vi "io.command-parser.AI.vi"(8 "error in":errorcluster, 10 "Reponse in":string="{ß\u0005\u0001\u0016\u0010\u0001\u0004\u0002ß}", 11 "IoConf in":T1={"ADDR"=0, "Label"="", "Type"=enum."DI", "Mode"=enum."RIO", "Value"="", "Tags"="", "calibration"=[]} {"calibration"."Y" format="%#.3f"; "calibration"."X" format="%#.3f"; "ADDR" format="%04d"}) -> (0 "error out":errorcluster, 1 "AI uncalib out":u16, 2 "AI out":dbl=1.0)   [LabVIEW 2024]
uses:
  controls/IONode.ctl
  controls/type.address.ctl
  controls/enum.io.type.ctl
  controls/enum.io.mode.ctl
  controls/typeXyPoint.ctl
panel:
  out "*(type *) &x 2":string
  out "*(type *) &x":u16
  # "\\DF\\05\\01\\16\\10\\01\\04\\02\\DF"
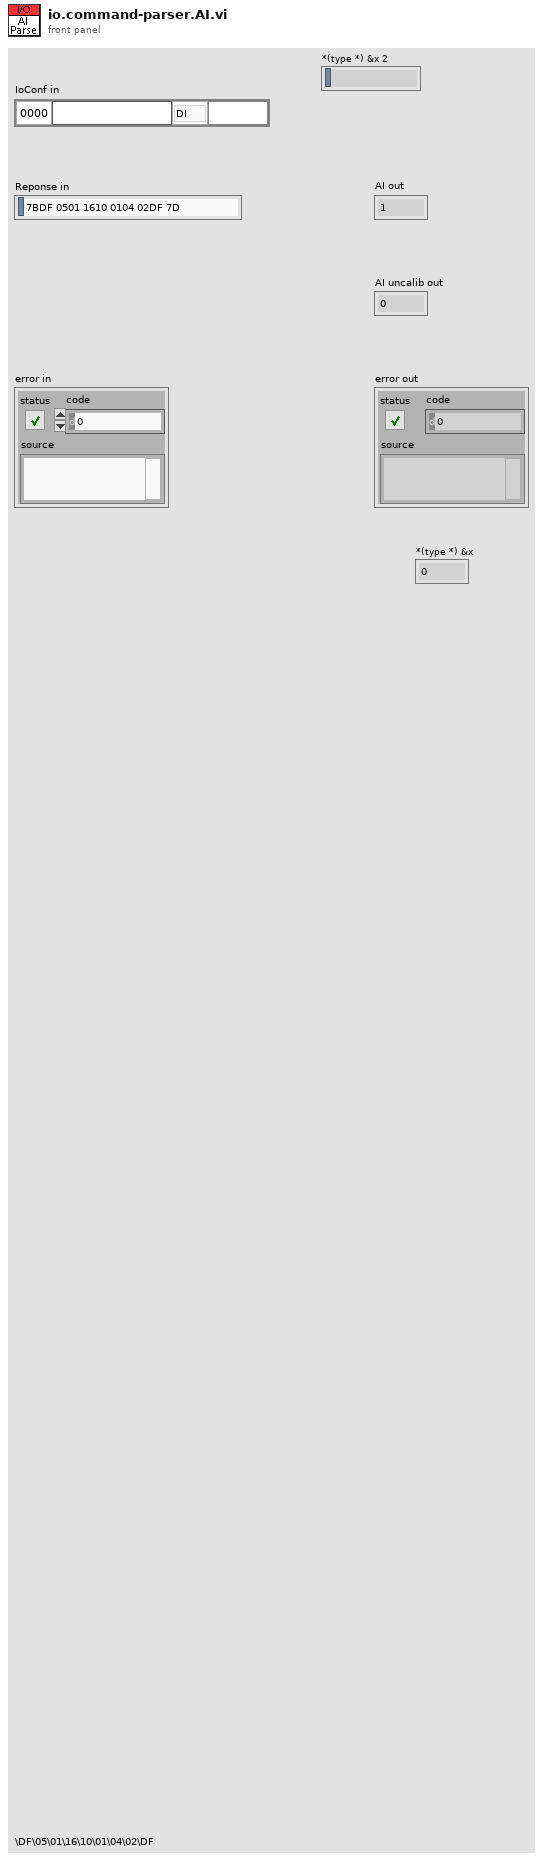
[diagram p1: front panel]
types:
  T1 = typedef "IONode.ctl" = cluster{"ADDR":T2, "Label":string, "Type":T3, "Mode":T4, "Value":string, "Tags":string, "calibration":T5[]}
  T2 = typedef "type.address.ctl" = u16
  T3 = typedef "enum.io.type.ctl" = enum16{"Type", "DI", "DO", "AI", "AO", "VL", "BUF"}
  T4 = typedef "enum.io.mode.ctl" = enum16{"Mode", "RIO", "SIM"}
  T5 = typedef "typeXyPoint.ctl" = cluster{"X":dbl, "Y":dbl}
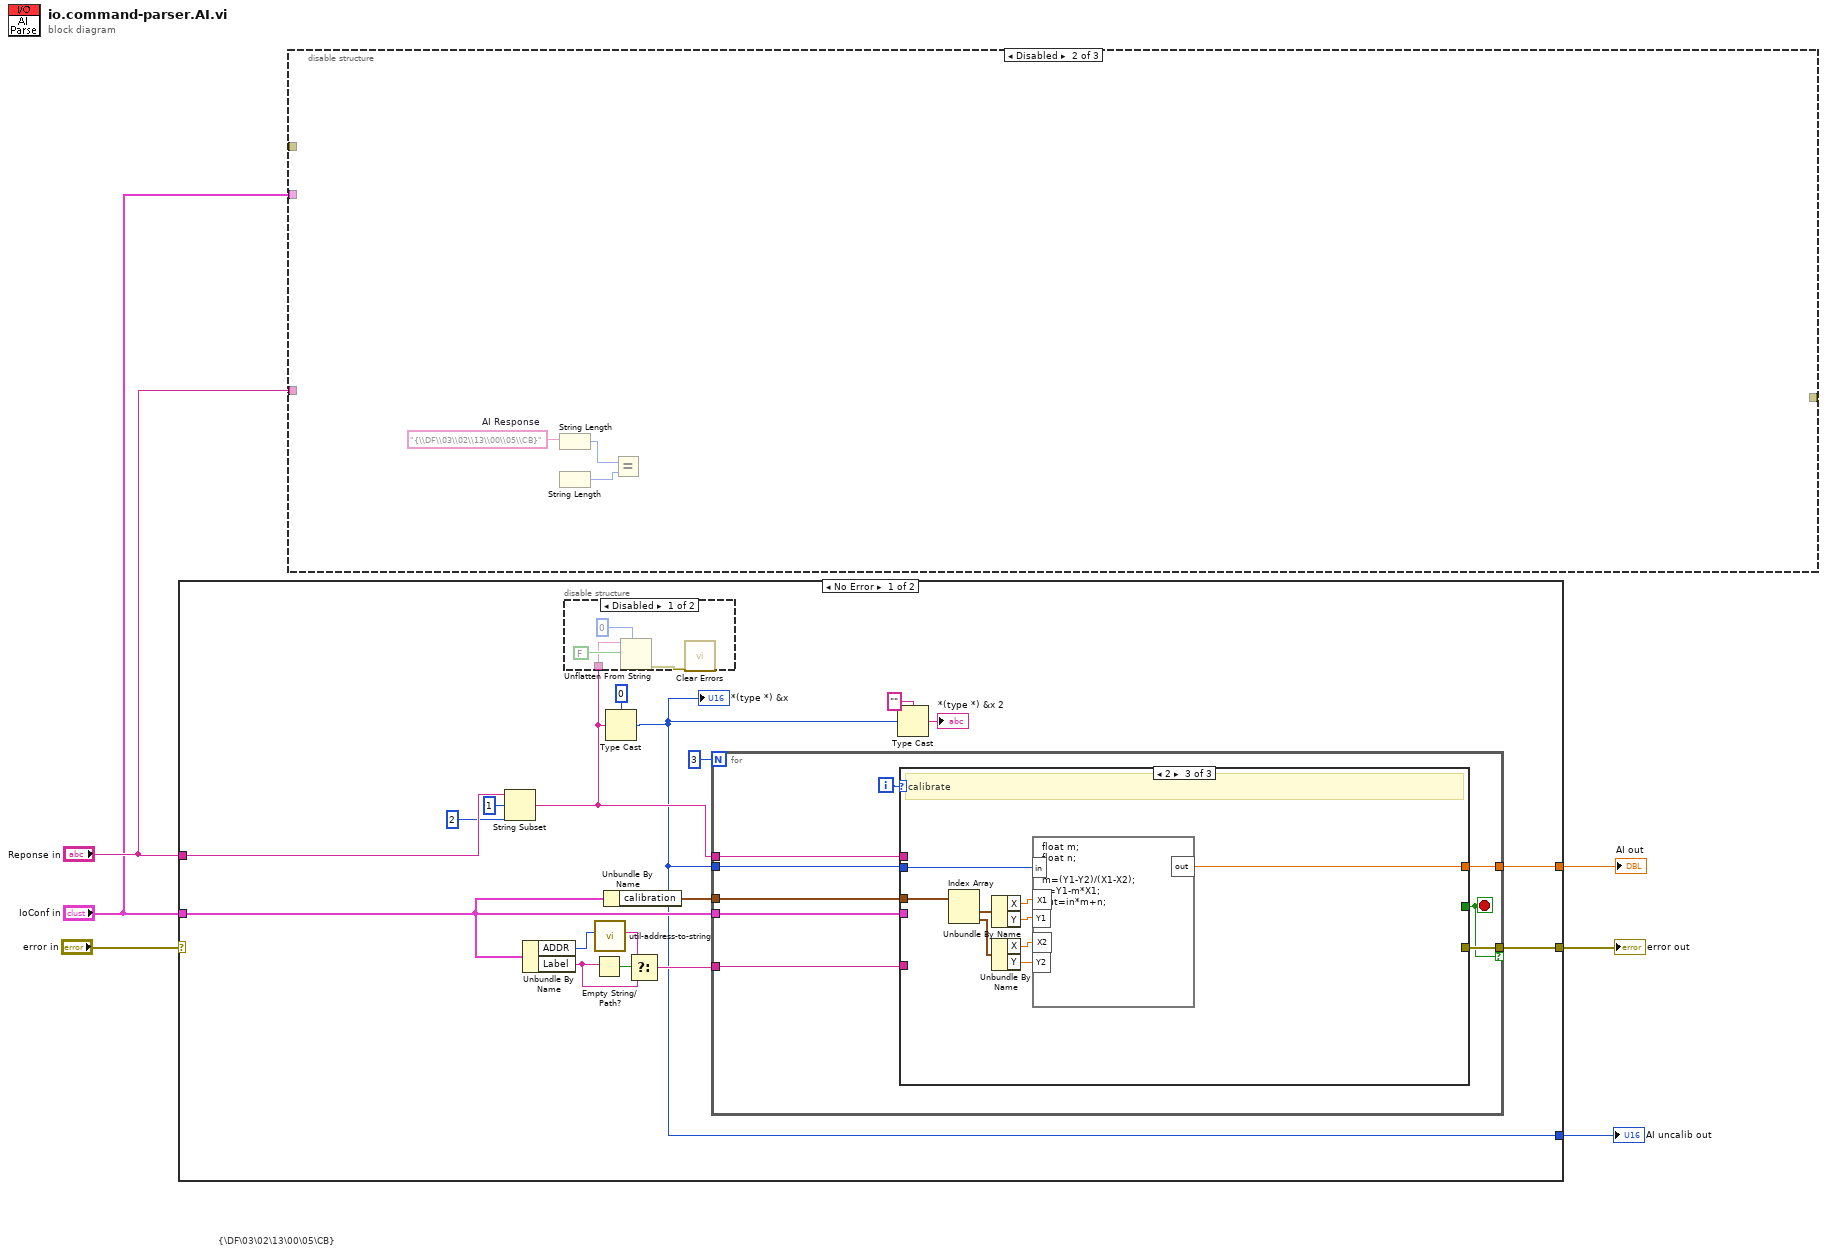
[diagram p0: block diagram]
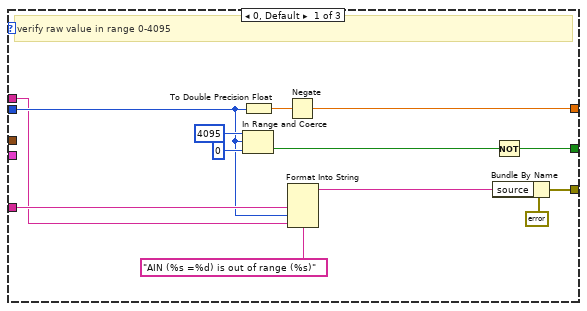
[diagram p3: hidden frame]
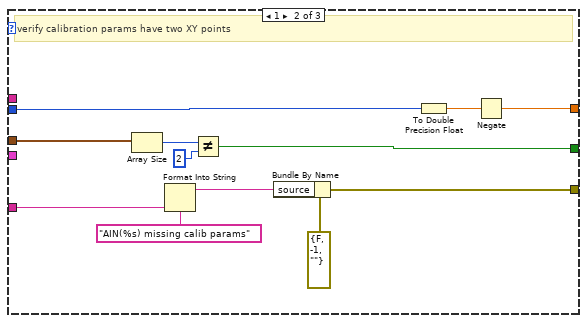
[diagram p4: hidden frame]
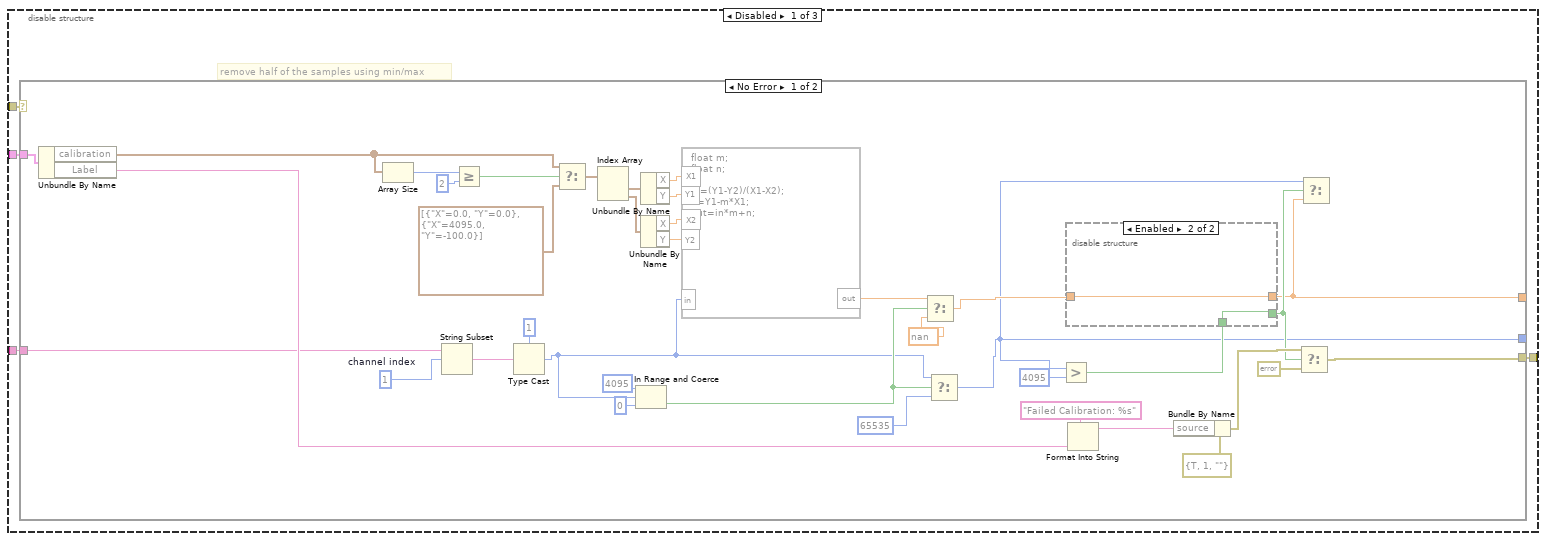
[diagram p6: hidden frame]
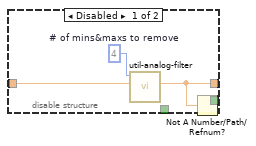
[diagram p7: hidden frame]
diagram:
  # "{\\DF\\03\\02\\13\\00\\05\\CB}"
  n1 = case shown="No Error" "error in" {
    selector: "error in" -> [_ w72]
    tunnel: "Reponse in" -> [w21 _]
    tunnel: "IoConf in" -> [w24 _]
    tunnel: [w23 _] -> w4
    tunnel: [w8 _] -> w3
    tunnel: [w22 w72] -> w2
    frame No Error {
      n2 = String Subset(string=w21, offset (0)=1, length (rest)=2 ("length (rest)")) -> (substring=w9:string)
      n3 = Unbundle By Name(w24) -> ("ADDR"=w19:T2, "Label"=w16:string)
      n4 = disable-structure shown="Disabled" {
        disable-tunnel: w9 -> [w25 _]
        frame Disabled {
          n5 = Unflatten From String(type=u16 0, binary string=w25, data includes array or string size? (T)=FALSE) -> (error out=w26:errorcluster)  [unwired: 2 in, 2 out]
          n6 = call <vilib>:"Clear Errors.vi"("error in (no error)"=w26) -> ()  [unwired: 5 in, 2 out]
        }
        frame Enabled {
        }
      }
      n7 = Empty String/Path?(string/path=w16) -> (empty?=w18:bool)
      n8 = call "util-address-to-string.vi"("ADDR"=w19) -> ("str(ADDR)"=w17:string)  [unwired: 10 in]
      n9 = Unbundle By Name(w24) -> ("calibration"=w13:T5[])
      n10 = Type Cast(type=u16 0, x=w9) -> (*(type *) &x=w8:u16)
      "*(type *) &x" <- w8
      n11 = Select(t=w17, s=w18, f=w16) -> (s? t:f=w15:string)
      n12 = for {
        N: 3 -> [_]
        tunnel: [w36] -> w22 if=w35
        tunnel: w24 -> [w34]
        tunnel: w15 -> [w33]
        tunnel: w8 -> [w32]
        tunnel: w13 -> [w31]
        tunnel: [w30] -> w23
        tunnel: w9 -> [w29]
        i -> [w37]
        stop <- w35 stop-if-true
        n13 = case shown="2" w37 {
          tunnel: [w47 w61 _] -> w35
          tunnel: [w43 w56 _] -> w36
          tunnel: w34 -> [_ _ _]
          tunnel: w33 -> [w42 w59 _]
          tunnel: w32 -> [w39 w51 w64]
          tunnel: w31 -> [_ w55 w65]
          tunnel: [w40 w53 w63] -> w30
          tunnel: w29 -> [w38 _ _]
          frame 0, Default {
            # "verify raw value in range 0-4095"
            n14 = In Range and Coerce(upper limit=u16 4095 ("lower limit"), x=w39, lower limit=u16 0) -> (In Range?=w48:bool)  [unwired: 1 out]
            n15 = To Double Precision Float(number=w39) -> (double precision float=w41:dbl)
            n16 = Negate(x=w41) -> (-x=w40:dbl)
            n17 = Format Into String(format string="AIN (%s =%d) is out of range (%s)", w42, w39, w38) -> (resulting string=w45:string)  [unwired: 2 in, 1 out]
            n18 = Bundle By Name(cluster=errorcluster {"status"=TRUE, "code"=-1, "source"=""} ("error constant"), "source"=w45) -> (w43:errorcluster)
            n19 = Not(x=w48) -> (.not. x?=w47:bool)
          }
          frame 1 {
            # "verify calibration params have two XY points"
            n20 = Array Size(array=w55) -> (size(s)=w52:i32)
            n21 = Format Into String(format string="AIN(%s) missing calib params", w59) -> (resulting string=w57:string)  [unwired: 2 in, 1 out]
            n22 = Not Equal?(x=w52, y=2) -> (x != y?=w61:bool)
            n23 = Bundle By Name(cluster=errorcluster {"status"=FALSE, "code"=-1, "source"=""} ("error constant"), "source"=w57) -> (w56:errorcluster)
            n24 = To Double Precision Float(number=w51) -> (double precision float=w54:dbl)
            n25 = Negate(x=w54) -> (-x=w53:dbl)
          }
          frame 2 {
            # "calibrate"
            n26 = Index Array(array=w65) -> (element #1=w67:T5, element #2=w66:T5)  [unwired: 2 in]
            n27 = Unbundle By Name(w67) -> ("X"=w71:dbl, "Y"=w69:dbl)
            n28 = Unbundle By Name(w66) -> ("X"=w70:dbl, "Y"=w68:dbl)
            n29 = formula code="float m;\nfloat n;\n\nm=(Y1-Y2)/(X1-X2);\nn=Y1-m*X1;\nout=in*m+n;"("Y1"=w69, "X1"=w71, "Y2"=w68, "X2"=w70, "in"=w64) -> ("out"=w63:dbl)
          }
        }
      }
      n30 = Type Cast(type="" ("match + rest of string"), x=w8) -> (*(type *) &x=→"*(type *) &x 2":string)
    }
    frame Error {
    }
  }
  "error out" <- w2
  "AI out" <- w4
  "AI uncalib out" <- w3
  n31 = disable-structure shown="Disabled" {
    disable-tunnel: _ -> [w76 _ _]
    disable-tunnel: [w75 _ _] -> _
    disable-tunnel: "Reponse in" -> [w74 _ _]
    disable-tunnel: "IoConf in" -> [w73 _ _]
    frame Disabled {
      # "remove half of the samples using min/max"
      n32 = case shown="No Error" w76 {
        selector: w76 -> [_ w120]
        tunnel: w73 -> [w113 _]
        tunnel: [w100 _] -> _
        tunnel: [w110 w120] -> w75
        tunnel: [w77 _] -> _
        tunnel: w74 -> [w81 _]
        frame No Error {
          w98 = 1  # channel index
          n33 = Unbundle By Name(w113) -> ("calibration"=w111:T5[], "Label"=w107:string)
          n34 = Array Size(array=w111) -> (size(s)=w90:i32)
          n35 = String Subset(string=w81, offset (0)=w98) -> (substring=w97:string)  [unwired: 1 in]
          n36 = Greater Or Equal?(x=w90, y=2) -> (x >= y?=w88:bool)
          n37 = Type Cast(type=u16 1, x=w97) -> (*(type *) &x=w78:u16)
          n38 = Select(t=w111, s=w88, f=T5[] [{"X"=0.0, "Y"=0.0}, {"X"=4095.0, "Y"=-100.0}]) -> (s? t:f=w87:T5[])
          n39 = Index Array(array=w87) -> (element #1=w95:T5, element #2=w96:T5)  [unwired: 2 in]
          n40 = In Range and Coerce(upper limit=u16 4095 ("lower limit"), x=w78, lower limit=u16 0) -> (In Range?=w80:bool)  [unwired: 1 out]
          n41 = Unbundle By Name(w95) -> ("X"=w91:dbl, "Y"=w93:dbl)
          n42 = Unbundle By Name(w96) -> ("X"=w92:dbl, "Y"=w94:dbl)
          n43 = formula code="float m;\nfloat n;\n\nm=(Y1-Y2)/(X1-X2);\nn=Y1-m*X1;\nout=in*m+n;"("Y1"=w93, "X1"=w91, "Y2"=w94, "X2"=w92, "in"=w78) -> ("out"=w82:dbl)
          n44 = Select(t=w82, s=w80, f=nan) -> (s? t:f=w112:dbl)
          n45 = Select(t=w78, s=w80, f=u16 65535) -> (s? t:f=w77:u16)
          n46 = Greater?(x=w77, y=u16 4095) -> (0:w101:bool)
          n47 = disable-structure shown="Enabled" {
            disable-tunnel: w112 -> [w117 w119]
            disable-tunnel: [w115 w118] -> w103
            disable-tunnel: [w114 w119] -> w100
            disable-tunnel: w101 -> [_ w118]
            frame Disabled {
              w116 = 4  # # of mins&maxs to remove
              n48 = call "util-analog-filter.vi"("Array"=w117, "# of mins&maxs to remove"=w116) -> ("Filtered Value"=w114:dbl)  [unwired: 9 in]
              n49 = Not A Number/Path/Refnum?(number/path/refnum=w114) -> (NaN/Path/Refnum?=w115:bool)
            }
            frame Enabled {
            }
          }
          n50 = Format Into String(format string="Failed Calibration: %s" ("source"), w107) -> (resulting string=w105:string)  [unwired: 2 in, 1 out]
          n51 = Bundle By Name(cluster=errorcluster {"status"=TRUE, "code"=1, "source"=""} ("error IO"), "source"=w105) -> (w104:errorcluster)
          n52 = Select(t=w104, s=w103, f=errorcluster {"status"=FALSE, "code"=0, "source"=""} ("error IO")) -> (s? t:f=w110:errorcluster)
          n53 = Select(t=w77, s=w103, f=w100) -> ()  [unwired: 1 out]
        }
        frame Error {
        }
      }
    }
    frame Disabled {
      w121 = "{\\DF\\03\\02\\13\\00\\05\\CB}"  # AI Response
      n54 = String Length(string=w121) -> (length=w122:i32)
      n55 = String Length() -> (length=w123:i32)  [unwired: 1 in]
      n56 = Equal?(x=w122, y=w123) -> ()  [unwired: 1 out]
    }
    frame Enabled {
    }
  }
